vi "check jsonrpc version.vi"(8 "error in (no error)":errorcluster, 11 "Request in":variant) -> (0 "error out":errorcluster, 3 "Request out":variant)   [LabVIEW 2017, in "JSONRPC Server.lvclass"]
uses:
  JSONRPC Server.lvclass
  <vilib>/National Instruments/Variant Data Manipulation/Variant Data Manipulation.lvlib
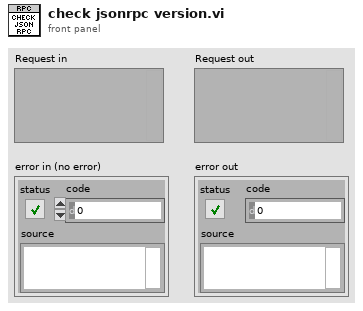
[diagram p1: front panel]
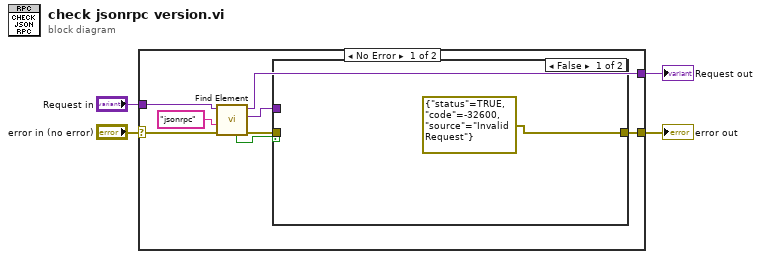
[diagram p0: block diagram]
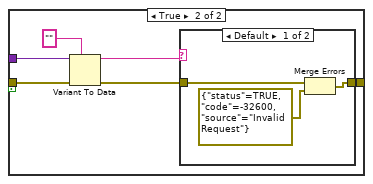
[diagram p2: hidden frame]
diagram:
  n1 = case shown="No Error" "error in (no error)" {
    selector: "error in (no error)" -> [w10 w24]
    tunnel: [w11 w25] -> w4
    tunnel: "Request in" -> [w9 w25]
    tunnel: [w7 w24] -> w1
    frame No Error {
      n2 = call <vilib>:"Find Element.vi"("error in (no error)"=w10, "Name"="jsonrpc", "Variant (Cluster) in"=w9) -> ("error out"=w8:errorcluster, "element"=w12:variant, "Variant (Cluster) out"=w11:variant, "found?"=w5:bool)  [unwired: 4 in, 1 out]
      n3 = case shown="False" w5 {
        tunnel: w12 -> [_ w19]
        tunnel: w8 -> [_ w17]
        tunnel: [errorcluster {"status"=TRUE, "code"=-32600, "source"="Invalid Request"} ("error out") w16] -> w7
        frame False {
        }
        frame True {
          n4 = Variant To Data(error in=w17, type="" ("Name"), Variant=w19) -> (data=w14:string, error out=w15:errorcluster)
          n5 = case shown="Default" w14 {
            tunnel: [w21 w23] -> w16
            tunnel: w15 -> [w20 w23]
            frame Default {
              n6 = Merge Errors(w20, errorcluster {"status"=TRUE, "code"=-32600, "source"="Invalid Request"} ("error out")) -> (w21:errorcluster)
            }
            frame "2.0" {
            }
          }
        }
      }
    }
    frame Error {
    }
  }
  "Request out" <- w4
  "error out" <- w1
